vi "DCM Get section.vi"(8 "error in":errorcluster, 10 "Label.Text in":string, 11 "Data in":T2 {"Device Ref" format="%.0x"; "Section Ref" format="%.0x"}) -> (0 "error out":errorcluster, 1 "Section Ptr":T1=18446744073709551615 format="%.0x", 3 "Data out":T2 {"Device Ref" format="%.0x"; "Section Ref" format="%.0x"})   [LabVIEW 2016, in "DCM System Explorer.lvlib"]
uses:
  DCM System Explorer.lvlib
  <vilib>/NI Veristand/Custom Device API/Custom Device Item Ref.ctl
  <vilib>/NI VeriStand/Custom Device API/Custom Device API.lvlib
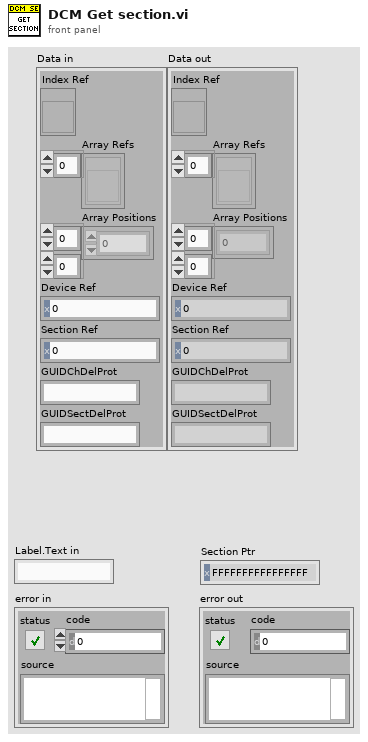
[diagram p1: front panel]
types:
  T1 = typedef "Custom Device API.lvlib/Custom Device Item Ref.ctl" = u64
  T2 = cluster{"Index Ref":refnum<vi>, "Array Refs":refnum<vi>[], "Array Positions":i32[][], "Device Ref":T1, "Section Ref":T1, "GUIDChDelProt":string, "GUIDSectDelProt":string}
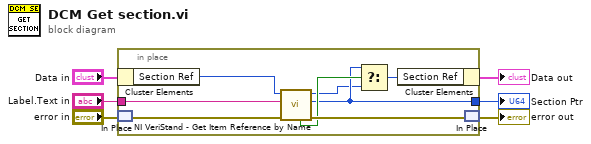
[diagram p0: block diagram]
diagram:
  n1 = in-place {
    in-place-border: "Label.Text in" -> [w13]
    in-place-border: [w8] -> w1
    n2 = in-place-cluster #1("Data in") -> ("Section Ref"=w14:T1)
    n3 = in-place-match #2("error in") -> (w12:errorcluster)
    n4 = call <vilib>:"NI VeriStand - Get Item Reference by Name.vi"("error in (no error)"=w12, "Item Name"=w13, "Parent Ref in"=w14) -> ("error out"=w11:errorcluster, "Item Ref"=w8:T1, "Parent Ref out"=w7:T1, "Found"=w9:bool)  [unwired: 5 in]
    n5 = Select(t=w8, s=w9, f=w7) -> (s? t:f=w10:T1)
    n6 = in-place-cluster #1("Section Ref"=w10) -> (→"Data out":T2)
    n7 = in-place-match #2(w11) -> (→"error out":errorcluster)
  }
  "Section Ptr" <- w1
